vi "U3 eDI Example.vi"() -> (0 "error out":errorcluster)   [LabVIEW 2021]
panel:
  out "State":bool
  in  "Channel":i32=4
  in  "FirstFound":bool=TRUE
  in  "Address":string="1"
  out "Error Message":string
  # "Reads 1 digital input using the UD easy function eDI."
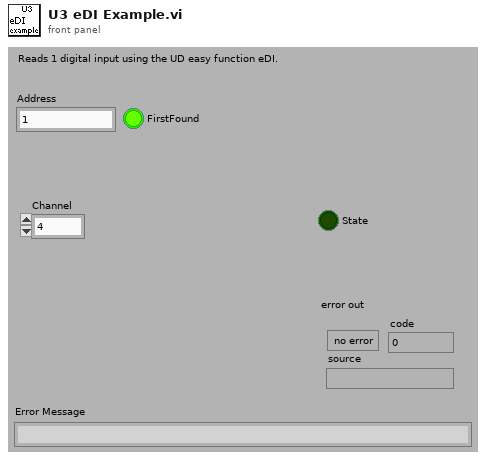
[diagram p1: front panel]
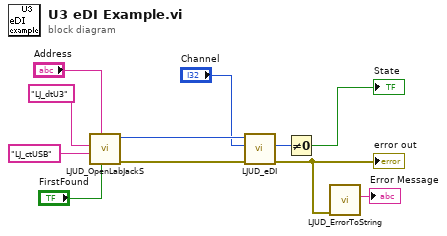
[diagram p0: block diagram]
diagram:
  n1 = call "LJUD_OpenLabJackS.vi"("FirstFound"="FirstFound", "Address"="Address", "ConnectionType"="LJ_ctUSB", "DeviceType"="LJ_dtU3") -> ("error out"=w5:errorcluster, "Handle"=w6:i32)  [unwired: 5 in, 1 out]
  n2 = call "LJUD_eDI.vi"("error in"=w5, "Channel"="Channel", "Handle In"=w6) -> ("error out"=w4:errorcluster, "State"=w2:i32)  [unwired: 6 in, 1 out]
  "error out" <- w4
  n3 = Not Equal To 0?(x=w2) -> (x != 0?=→"State":bool)
  n4 = call "LJUD_ErrorToString.vi"("error in"=w4) -> ("String"=→"Error Message":string)  [unwired: 10 in]
